vi "AnalyzeVIs.vi"(8 "error in (no error)":errorcluster, 11 "VIs":refnum<vi>[](array[refnum])) -> (0 "error out":errorcluster, 2 "VIsData":T1[](array[typedef]), 3 "VIs out":refnum<vi>[](array[refnum]))   [LabVIEW 2020]
uses:
  _controls/_VIWiresData.ctl
panel:
  in  "Stop Button":bool
  out "Progress":dbl(slide) caption="Analyzing..." scale=0.0..1.0
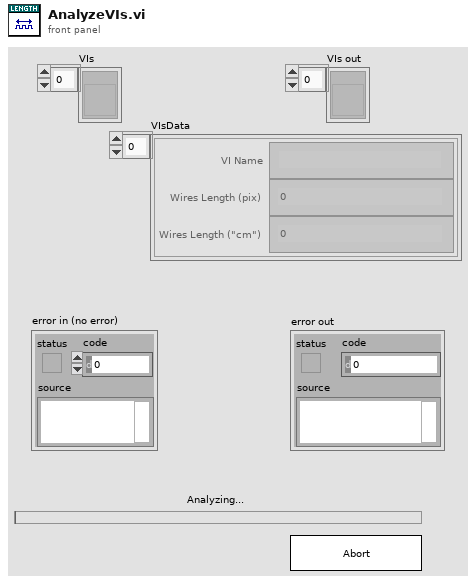
[diagram p1: front panel]
types:
  T1 = typedef "_VIWiresData.ctl" = cluster{"VI Name":string, "Wires Length (pix)":dbl, "Wires Length (\"cm\")":dbl}
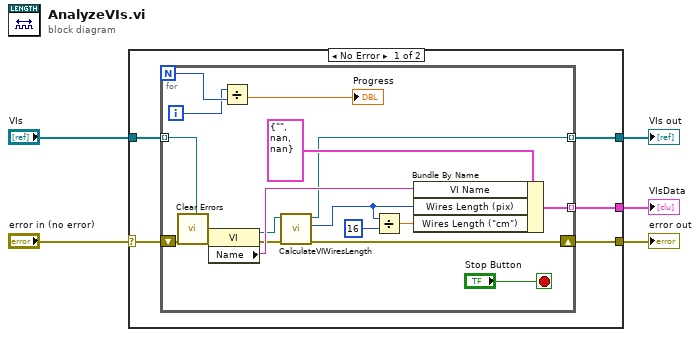
[diagram p0: block diagram]
diagram:
  n1 = case shown="No Error" "error in (no error)" {
    selector: "error in (no error)" -> [w9 w29]
    tunnel: [w8 w29] -> w5
    tunnel: [w7 w28] -> w3
    tunnel: "VIs" -> [w10 w28]
    tunnel: [w6 _] -> w1
    frame No Error {
      n2 = for {
        N -> [w14]
        tunnel: w10 -> [w26] mode=indexing
        shift-right: [w20] -> w8
        shift-left: w9 -> [w27]
        tunnel: [w19] -> w7 mode=indexing
        tunnel: [w23] -> w6 mode=indexing
        i -> [w13]
        stop <- "Stop Button" stop-if-true
        n3 = call <vilib>:"Clear Errors.vi"("error in (no error)"=w27) -> ("error out"=w11:errorcluster)  [unwired: 5 in, 1 out]
        n4 = property class="VI"(reference=w26, error in=w11) -> (reference out=w22:refnum<vi>, error out=w21:errorcluster, "Name"=w24:string)
        n5 = Divide(x=w13, y=w14) -> (x/y=→"Progress":dbl)
        n6 = call "CalculateVIWiresLength.vi"("error in (no error)"=w21, "VI Refnum"=w22) -> ("error out"=w20:errorcluster, "WiresDistance"=w18:i32, "VI Refnum out"=w19:refnum<vi>)  [unwired: 7 in]
        n7 = Divide(x=w18, y=i16 16) -> (x/y=w17:dbl)
        n8 = Bundle By Name(cluster=T1 {"VI Name"="", "Wires Length (pix)"=nan, "Wires Length (\"cm\")"=nan} ("VIWiresData"), "VI Name"=w24, "Wires Length (pix)"=w18, "Wires Length (\"cm\")"=w17) -> (w23:T1)
      }
    }
    frame Error {
    }
  }
  "error out" <- w5
  "VIs out" <- w3
  "VIsData" <- w1
